vi "From TCP Async.vi"(8 "URI":refnum<class "URI.lvclass">, 9 "TCP":refnum<k5>, 10 "Server Endpoint":refnum<class "Endpoint.lvclass">, 11 "Listener Notifier":refnum<notifier>) -> ()   [LabVIEW 2020, in "Stream-Websocket.lvlib" / "Websocket Client.lvclass"]
uses:
  Websocket Client.lvclass
  lv-stream/stream/Endpoint/Endpoint.lvclass
  Listener Status.ctl
  Stream-Websocket.lvlib
  lv-stream/stream/Connection State.ctl
  lv-stream/stream/Stream.lvlib
  lv-stream/stream/Connection/Connection.lvclass
  Listener Result.ctl
  lv-stream/stream/URI/URI.lvclass
panel:
  out "Client URI":string
  out "Server URI":string
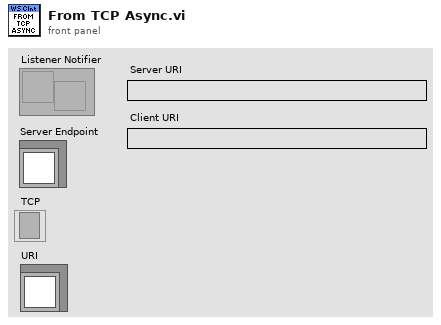
[diagram p1: front panel]
types:
  T1 = typedef "Stream-Websocket.lvlib/Listener Status.ctl" = enum16{"Successful", "Unsuccessful"}
  T2 = typedef "Stream-Websocket.lvlib/Listener Result.ctl" = cluster{"Status":T1, "Client":refnum<class "Websocket Client.lvclass">}
  T3 = typedef "Stream.lvlib/Connection State.ctl" = enum16{"Connected", "Disconnected"}
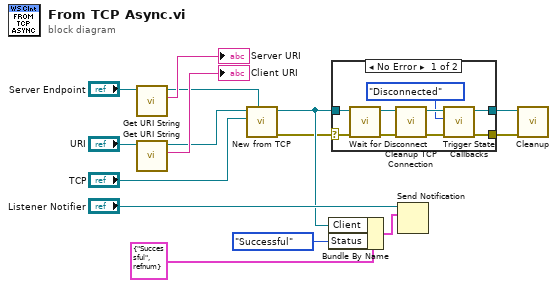
[diagram p0: block diagram]
diagram:
  n1 = call "Get URI String.vi"("Endpoint in"="Server Endpoint") -> ("URI String"=→"Server URI":string, "Endpoint out"=w2:refnum<class "Endpoint.lvclass">)  [unwired: 8 in, 1 out]
  n2 = call "Get URI String.vi"("URI in"="URI") -> ("URI String"=→"Client URI":string, "URI out"=w1:refnum<class "URI.lvclass">)  [unwired: 8 in, 1 out]
  n3 = call "New from TCP.vi"("From"=w2, "TCP Connection"="TCP", "URI"=w1) -> ("error out"=w4:errorcluster, "Client"=w8:refnum<class "Websocket Client.lvclass">)  [unwired: 7 in]
  n4 = Bundle By Name(cluster=T2 {"Status"=enum."Successful", "Client"=refnum} ("Listener Result"), "Client"=w8, "Status"=Listener_Status."Successful") -> (w11:T2)
  n5 = case shown="No Error" w4 {
    selector: w4 -> [w24 w26]
    tunnel: w8 -> [w23 w25]
    tunnel: [w17 w25] -> w10
    tunnel: [w16 w26] -> w9
    frame No Error {
      n6 = call "Wait for Disconnect.vi"("error in (no error)"=w24, "Websocket Client in"=w23) -> ("error out"=w21:errorcluster, "Websocket Client out"=w22:refnum<class "Websocket Client.lvclass">)  [unwired: 8 in]
      n7 = call "Cleanup TCP Connection.vi"("error in (no error)"=w21, "Websocket Client in"=w22) -> ("error out"=w19:errorcluster, "Websocket Client out"=w20:refnum<class "Websocket Client.lvclass">)  [unwired: 8 in]
      n8 = call "Trigger State Callbacks.vi"("error in (no error)"=w19, "State"=Connection_State."Disconnected", "Connection in"=w20) -> ("error out"=w16:errorcluster, "Connection out"=w17:refnum<class "Websocket Client.lvclass">)  [unwired: 7 in]
    }
    frame Error {
    }
  }
  n9 = Send Notification(notification=w11, notifier="Listener Notifier") -> ()  [unwired: 1 in, 2 out]
  n10 = call-dynamic "Cleanup.vi"("error in (no error)"=w9, "Websocket Client in"=w10) -> ()  [unwired: 9 in, 1 out]
